vi "CMC_Homework_01.vi"() -> ()   [LabVIEW 2013]
panel:
  in  "stop":bool
  out "Color Box":u32(colorbox)
  in  "Green":i32(slide) min=0 step=1 scale=0.0..255.0
  in  "Blue":i32(slide) min=0 step=1 scale=0.0..255.0
  in  "Red":i32(slide) min=0 step=1 scale=0.0..255.0
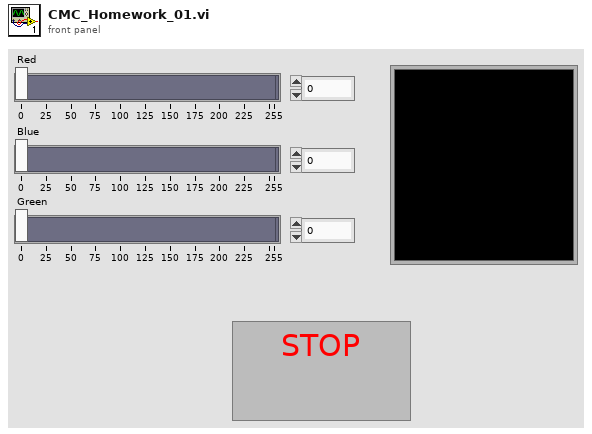
[diagram p1: front panel]
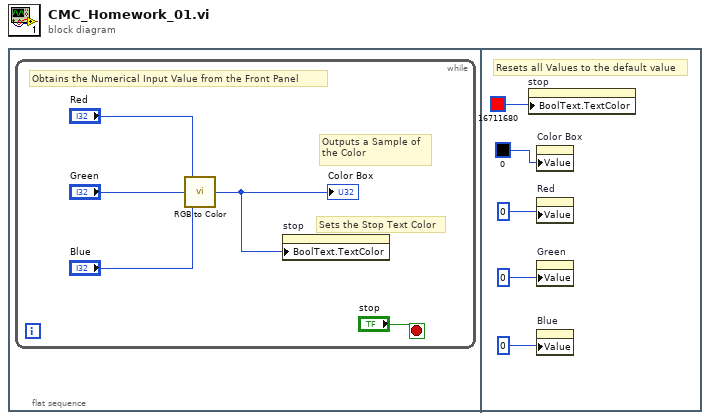
[diagram p0: block diagram]
diagram:
  n1 = flat-sequence {
    frame #0 {
      n2 = while {
        stop <- "stop" stop-if-true
        # "Sets the Stop Text Color"
        # "Outputs a Sample of\nthe Color"
        # "Obtains the Numerical Input Value from the Front Panel"
        n3 = call <vilib>:"RGB to Color.vi"("B"="Blue", "G"="Green", "R"="Red") -> ("Color"=w1:u32)
        "Color Box" <- w1
        n4 = property on="stop" class="Bool"("BoolText.TextColor"=w1) -> ()  [unwired: 2 in, 2 out]
      }
    }
    frame #1 {
      # "Resets all Values to the default value"
      n5 = property on="stop" class="Bool"("BoolText.TextColor"=u32 16711680) -> ()  [unwired: 2 in, 2 out]
      n6 = property on="Color Box" class="ColBox"("Value"=u32 0) -> ()  [unwired: 2 in, 2 out]
      n7 = property on="Red" class="Slide (strict)"("Value"=0) -> ()  [unwired: 2 in, 2 out]
      n8 = property on="Green" class="Slide (strict)"("Value"=0) -> ()  [unwired: 2 in, 2 out]
      n9 = property on="Blue" class="Slide (strict)"("Value"=0) -> ()  [unwired: 2 in, 2 out]
    }
  }
